vi "Configure_Tracker.vi"() -> ()   [LabVIEW 2011]
panel:
  out "Output":string[][](array[string])
  in  "PORT NAME":string="Inlet_Heaters"
  in  "Desired Address":i32
  in  "Current Address":i32
  # "Response"
  # "Comment"
  # "Command"
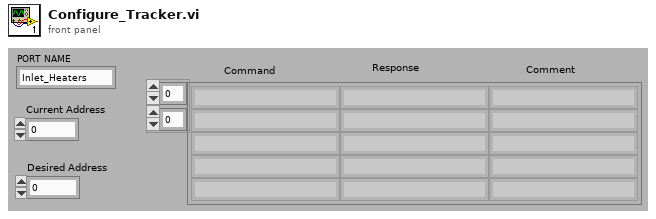
[diagram p1: front panel]
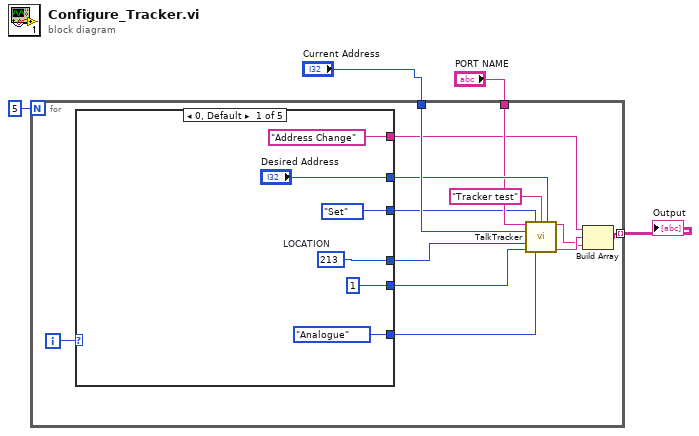
[diagram p0: block diagram]
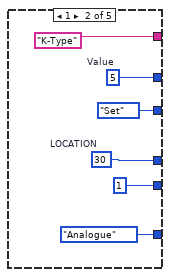
[diagram p2: hidden frame]
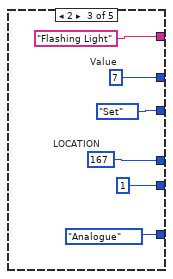
[diagram p3: hidden frame]
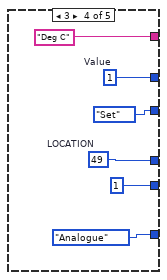
[diagram p4: hidden frame]
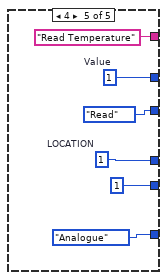
[diagram p5: hidden frame]
diagram:
  n1 = for {
    N: 5 -> [_]
    tunnel: "Current Address" -> [w16]
    tunnel: "PORT NAME" -> [w14]
    tunnel: [w10] -> w1 mode=indexing
    i -> [w17]
    n2 = case shown="0, Default" w17 {
      tunnel: ["Desired Address" w27 w33 w39 w45] -> w15
      tunnel: [w22 w29 w35 w41 w47] -> w13
      tunnel: [1 ("NO. LOCATIONS") 1 ("NO. LOCATIONS") 1 ("NO. LOCATIONS") 1 ("NO. LOCATIONS") 1 ("NO. LOCATIONS")] -> w12
      tunnel: ["Address Change" "K-Type" "Flashing Light" "Deg C" "Read Temperature"] -> w11
      tunnel: [enum16{"Logic", "Analogue"}."Analogue" ("Analogue") enum16{"Logic", "Analogue"}."Analogue" ("Analogue") enum16{"Logic", "Analogue"}."Analogue" ("Analogue") enum16{"Logic", "Analogue"}."Analogue" ("Analogue") enum16{"Logic", "Analogue"}."Analogue" ("Analogue")] -> w9
      tunnel: [enum16{"Set", "Read"}."Set" ("Set") enum16{"Set", "Read"}."Set" ("Set") enum16{"Set", "Read"}."Set" ("Set") enum16{"Set", "Read"}."Set" ("Set") enum16{"Set", "Read"}."Read" ("Set")] -> w8
      frame 0, Default {
        w22 = 213  # LOCATION
      }
      frame 1 {
        w27 = 5  # Value
        w29 = 30  # LOCATION
      }
      frame 2 {
        w33 = 7  # Value
        w35 = 167  # LOCATION
      }
      frame 3 {
        w39 = 1  # Value
        w41 = 49  # LOCATION
      }
      frame 4 {
        w45 = 1  # Value
        w47 = 1  # LOCATION
      }
    }
    n3 = call "TalkTracker.vi"("PORT NAME"=w14, "Set"=w8, "Channel Name"="Tracker test", "Value to set"=w15, "MODULE ADDRESS"=w16, "LOCATION"=w13, "NO. LOCATIONS"=w12, "Analogue"=w9) -> ("Response"=w5:string, "Comment out"=w6:string)  [unwired: 5 in, 1 out]
    n4 = Build Array(w11, w6, w5) -> (w10:string[])
  }
  "Output" <- w1
